vi "圓形ROI.vi"() -> ()   [LabVIEW 2015]
uses:
  <vilib>/Analysis/coordinate.llb/2D Cartesian Coordinate Rotation (Scalar).vi
  <vilib>/Analysis/NI_AALPro.lvlib
panel:
  in  "GAP":dbl
  out "Image":T1(plugin-control)
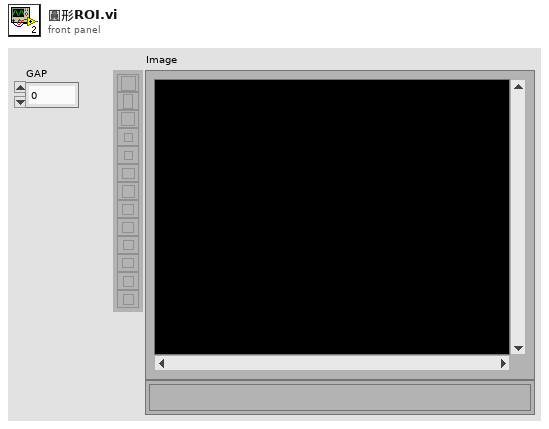
[diagram p1: front panel]
types:
  T1 = typedef "IMAQ Image.ctl" = refnum<image>
  T2 = cluster{"Global Rectangle":i32[], "Contours":cluster{"Contour Type":u32, "ROI Type":u32, "Points":i32[]}[]}
  T3 = typedef "IMAQ Circle" = cluster{"Center X":i32, "Center Y":i32, "Inner Radius":i32, "Outer Radius":i32, "Start Angle":dbl, "End Angle":dbl}
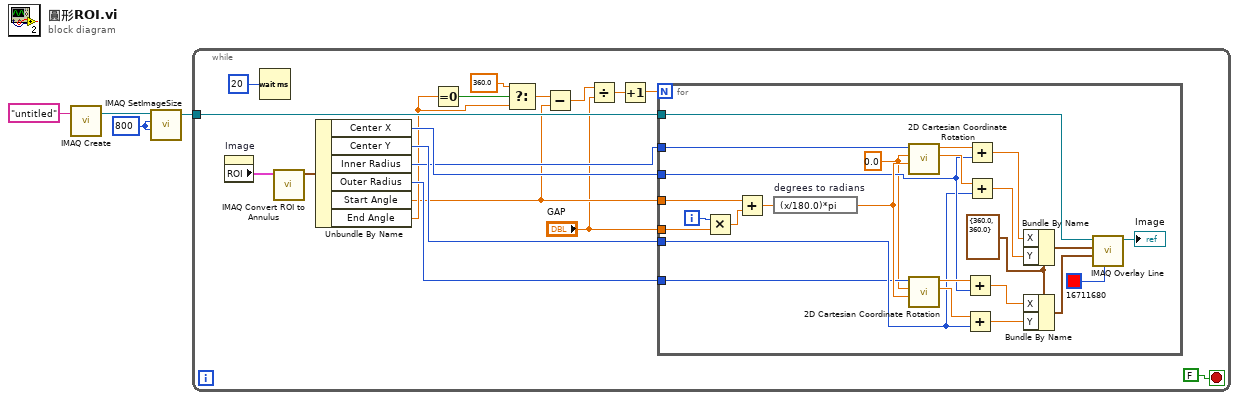
[diagram p0: block diagram]
diagram:
  w3 = 800 ("X Resolution")
  n1 = call "IMAQ Create"("Image Name"="untitled") -> ("New Image"=w4:T1)  [unwired: 4 in, 1 out]
  n2 = call "IMAQ SetImageSize"("Y Resolution"=w3, "X Resolution"=w3, "Image"=w4) -> ("Image Out"=w1:T1)  [unwired: 2 in, 1 out]
  n3 = while {
    tunnel: w1 -> [w21]
    stop <- FALSE stop-if-true
    n4 = property on="Image" class="ImageControl"() -> ("ROI"=w16:T2)  [unwired: 2 in, 2 out]
    n5 = Wait (ms)(milliseconds to wait=u32 20) -> ()  [unwired: 1 out]
    n6 = call "IMAQ Convert ROI to Annulus"("ROI Descriptor"=w16) -> ("Annulus"=w6:T3)  [unwired: 8 in, 1 out]
    n7 = Unbundle By Name(w6) -> ("Center X"=w20:i32, "Center Y"=w19:i32, "Inner Radius"=w18:i32, "Outer Radius"=w17:i32, "Start Angle"=w11:dbl, "End Angle"=w13:dbl)
    n8 = Equal To 0?(x=w13) -> (x = 0?=w15:bool)
    n9 = Select(t=360.0, s=w15, f=w13) -> (s? t:f=w12:dbl)
    n10 = Subtract(x=w12, y=w11) -> (x-y=w10:dbl)
    n11 = Divide(x=w10, y="GAP") -> (x/y=w8:dbl)
    n12 = Increment(x=w8) -> (x+1=w7:dbl)
    n13 = for {
      N: w7 -> [_]
      tunnel: w21 -> [w34]
      tunnel: w20 -> [w33]
      tunnel: w19 -> [w32]
      tunnel: w18 -> [w31]
      tunnel: w17 -> [w30]
      tunnel: "GAP" -> [w27]
      tunnel: w11 -> [w26]
      i -> [w28]
      w23 = cluster{"X":dbl, "Y":dbl} {"X"=360.0, "Y"=360.0}
      w29 = 0.0 ("y")
      n14 = Multiply(x=w28, y=w27) -> (x*y=w25:dbl)
      n15 = Add(x=w26, y=w25) -> (x+y=w24:dbl)
      n16 = expression code="(x/180.0)*pi" "degrees to radians"(w24) -> (w35:dbl)
      n17 = call-poly <vilib>:"2D Cartesian Coordinate Rotation.vi"("theta"=w35, "y"=w29, "x"=w31) -> ("y out"=w44:dbl, "x out"=w45:dbl)  [unwired: 6 in, 1 out]
      n18 = call-poly <vilib>:"2D Cartesian Coordinate Rotation.vi"("theta"=w35, "y"=w29, "x"=w30) -> ("y out"=w39:dbl, "x out"=w38:dbl)  [unwired: 6 in, 1 out]
      n19 = Add(x=w38, y=w33) -> (x+y=w37:dbl)
      n20 = Add(x=w39, y=w32) -> (x+y=w36:dbl)
      n21 = Add(x=w45, y=w33) -> (x+y=w43:dbl)
      n22 = Add(x=w44, y=w32) -> (x+y=w42:dbl)
      n23 = Bundle By Name(cluster=w23, "X"=w43, "Y"=w42) -> (w40:cluster{"X":dbl, "Y":dbl})
      n24 = Bundle By Name(cluster=w23, "X"=w37, "Y"=w36) -> (w41:cluster{"X":dbl, "Y":dbl})
      n25 = call "IMAQ Overlay Line"("Color"=u32 16711680, "End Point"=w41, "Start Point"=w40, "Image"=w34) -> ("Image Out"=→"Image":T1)  [unwired: 6 in, 1 out]
    }
  }
